vi "cdex - Initialize quadcopter 3D Model.vi"(8 "error in (no error)":errorcluster) -> (0 "error out":errorcluster, 3 "Main Scene Object":refnum<vi>)   [LabVIEW 2015]
uses:
  <vilib>/picture/3D Picture Control/Object/Create Object (drawable).vi
  <vilib>/picture/3D Picture Control/Object/Create Object (name).vi
  <vilib>/picture/3D Picture Control/Helpers/Apply Texture (no reference).vi
  <vilib>/picture/3D Picture Control/Object/Add Object (no reference).vi
  <vilib>/picture/3D Picture Control/Helpers/Set Clip Plane (no reference).vi
  <vilib>/picture/3D Picture Control/NI_3D Picture Control.lvlib
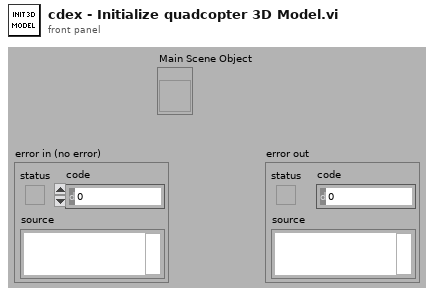
[diagram p1: front panel]
types:
  T1 = enum16{"As a Decal", "With Modulation", "With Blending", "As a replacement"}
  T2 = enum16{"Inherit Value", "No Culling", "Cull Back Face", "Cull Front Face", "Cull Both Faces"}
  T3 = enum16{"Normal Bin", "Opaque Bin", "Transparent Bin"}
  T4 = typedef "imagedata.ctl" = cluster{"image type":i32, "image depth":i32, "image":u8[], "mask":u8[], "colors":u32[], "Rectangle":cluster{"left":i16, "top":i16, "right":i16, "bottom":i16}}
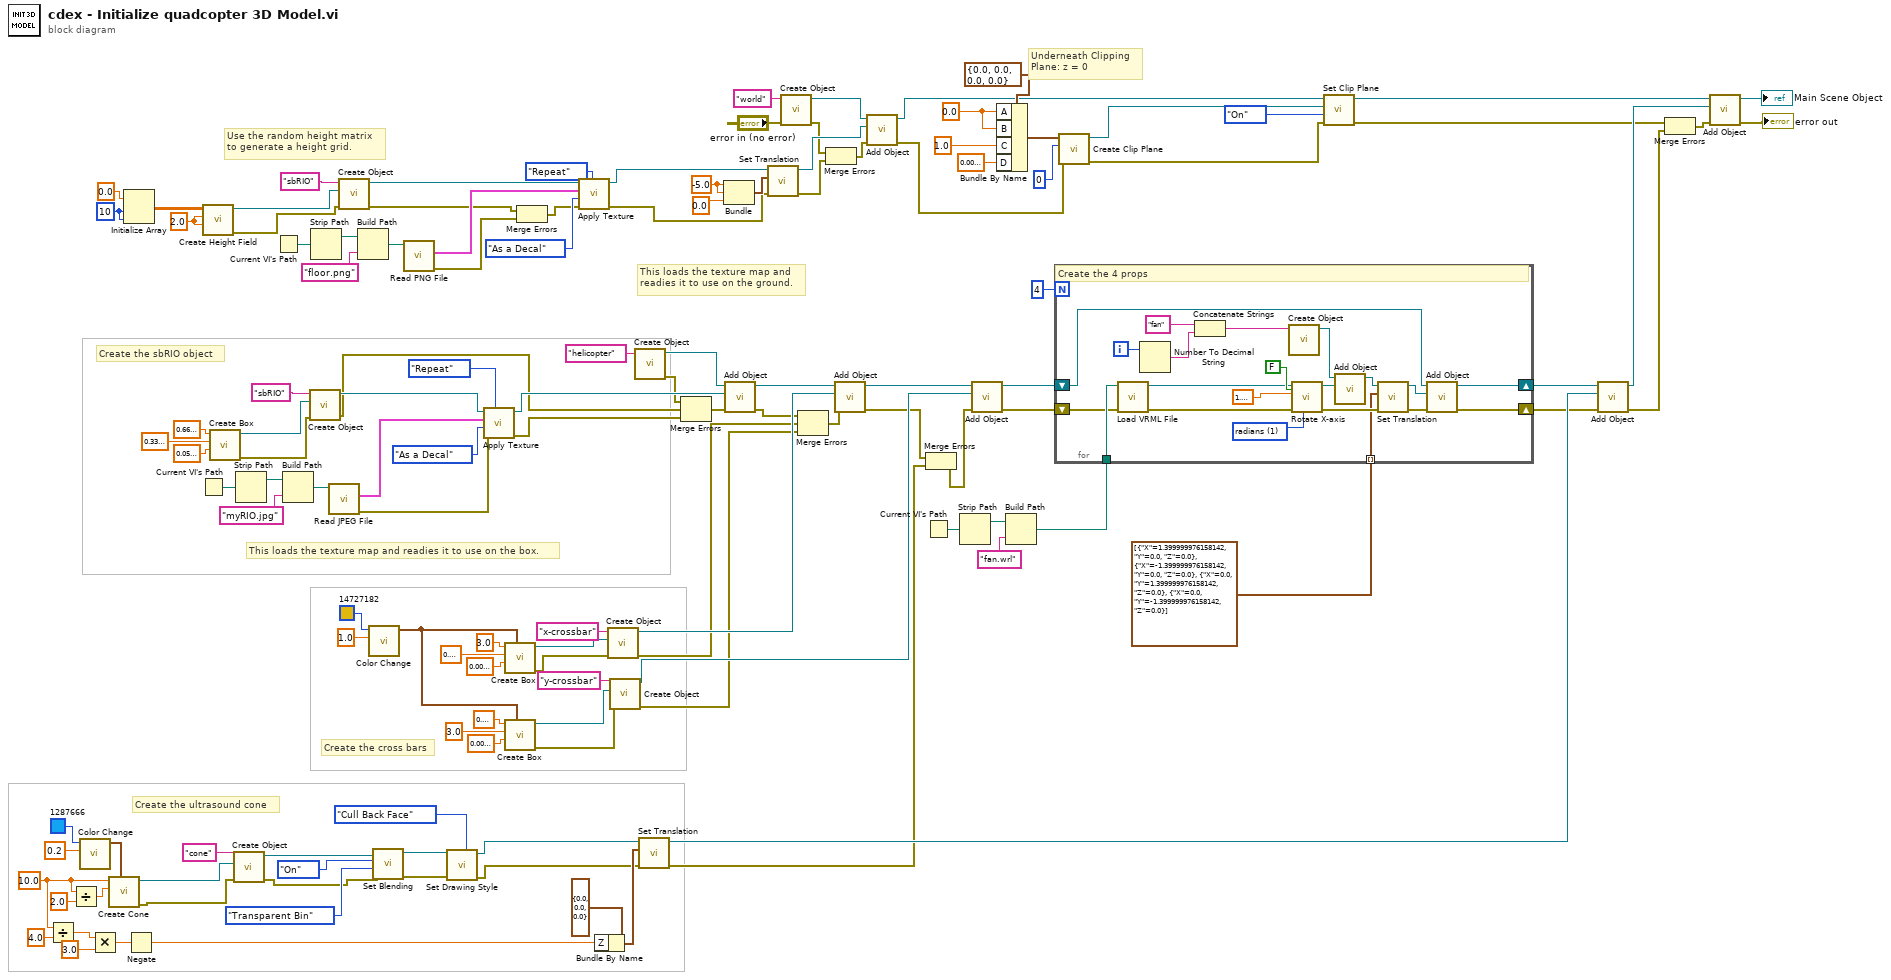
[diagram p0: block diagram]
diagram:
  w85 = 10 ("dimension size")
  w99 = sgl 0.0 ("A")
  w121 = sgl 10.0 ("Radius")
  w105 = sgl -5.0 ("y")
  w131 = sgl 2.0 ("Row Interval")
  # "This loads the texture map and\nreadies it to use on the ground."
  # "Underneath Clipping\nPlane: z = 0"
  # "Create the ultrasound cone"
  # "Create the cross bars"
  # "Create the sbRIO object"
  # "This loads the texture map and readies it to use on the box."
  # "Use the random height matrix\nto generate a height grid."
  n1 = Divide(x=w121, y=sgl 4.0) -> (x/y=w126:sgl)
  n2 = Divide(x=w121, y=sgl 2.0) -> (x/y=w122:sgl)
  n3 = call <vilib>:"Color Change.vi"("Alpha"=0.2, "Color"=u32 1287666) -> ("RGBA"=w118:cluster{"R":sgl, "G":sgl, "B":sgl, "A":sgl})  [unwired: 9 out]
  n4 = Multiply(x=w126, y=sgl 3.0) -> (x*y=w124:sgl)
  n5 = call <vilib>:"Create Cone.vi"("Color"=w118, "Radius"=w122, "Height"=w121) -> ("error out"=w44:errorcluster, "New Cone Refnum"=w64:refnum<vi>)  [unwired: 1 in, 6 out]
  n6 = Initialize Array(0.0 ("element"), w85, w85) -> (w83:dbl[][])
  n7 = Negate(x=w124) -> (-x=w128:sgl)
  n8 = Current VI's Path() -> (path=w104:path)
  n9 = call <vilib>:"Create Height Field.vi"("Column Interval"=w131, "Row Interval"=w131, "Data"=w83) -> ("error out"=w5:errorcluster, "New Height Field Refnum"=w56:refnum<vi>)  [unwired: 1 in, 6 out]
  n10 = call <vilib>:"Create Box.vi"("Length Z"=sgl 0.05, "Length Y"=sgl 0.33, "Length X"=sgl 0.66) -> ("error out"=w38:errorcluster, "New Box Refnum"=w78:refnum<vi>)  [unwired: 1 in, 6 out]
  n11 = call-poly <vilib>:"Create Object.vi"("error in (no error)"=w44, "Geometry"=w64, "Name"="cone") -> ("error out"=w43:errorcluster, "Scene:New Object"=w48:refnum<vi>)  [unwired: 7 in]
  n12 = Strip Path(path=w104) -> (stripped path=w103:path)  [unwired: 1 out]
  n13 = Current VI's Path() -> (path=w91:path)
  n14 = Build Path(base path=w103, name or relative path="myRIO.jpg") -> (appended path=w101:path)
  n15 = call-poly <vilib>:"Create Object.vi"("error in (no error)"=w38, "Geometry"=w78, "Name"="sbRIO") -> ("error out"=w35:errorcluster, "Scene:New Object"=w76:refnum<vi>)  [unwired: 7 in]
  n16 = Strip Path(path=w91) -> (stripped path=w92:path)  [unwired: 1 out]
  n17 = call <vilib>:"Read JPEG File.vi"("path to JPEG file"=w101) -> ("error out"=w37:errorcluster, "image data"=w72:T4)  [unwired: 1 in, 8 out]
  n18 = call-poly <vilib>:"Create Object.vi"("error in (no error)"=w5, "Geometry"=w56, "Name"="sbRIO") -> ("error out"=w6:errorcluster, "Scene:New Object"=w59:refnum<vi>)  [unwired: 7 in]
  n19 = Build Path(base path=w92, name or relative path="floor.png") -> (appended path=w94:path)
  n20 = call <vilib>:"Color Change.vi"("Alpha"=1.0, "Color"=u32 14727182) -> ("RGBA"=w100:cluster{"R":sgl, "G":sgl, "B":sgl, "A":sgl})  [unwired: 9 out]
  n21 = call <vilib>:"Set Blending.vi"("error in (no error)"=w43, "Bin"=T3."Transparent Bin" ("Blending:Bin"), "Mode"=enum16{"Inherit Value", "Off", "On"}."On" ("Blending:Mode"), "Scene Object In"=w48) -> ("error out"=w42:errorcluster, "Scene Object Out"=w47:refnum<vi>)  [unwired: 6 in]
  n22 = call <vilib>:"Read PNG File.vi"("path to PNG file"=w94) -> ("error out"=w8:errorcluster, "image data"=w57:T4)  [unwired: 1 in, 8 out]
  n23 = call <vilib>:"Set Drawing Style.vi"("Face Culling Mode"=T2."Cull Back Face" ("Draw Style:Face Culling Mode"), "error in (no error)"=w42, "Scene Object In"=w47) -> ("error out"=w41:errorcluster, "Scene Object Out"=w45:refnum<vi>)  [unwired: 7 in]
  n24 = call-poly <vilib>:"Apply Texture.vi"("Horizontal Wrap Mode"=enum16{"Clamp", "Repeat"}."Repeat", "error in (no error)"=w37, "Apply Mode"=T1."As a Decal", "Image Data"=w72, "Scene Object In"=w76) -> ("error out"=w36:errorcluster, "Scene Object Out"=w75:refnum<vi>)  [unwired: 5 in]
  n25 = call <vilib>:"Create Box.vi"("Color"=w100, "Length Z"=sgl 0.01, "Length Y"=sgl 0.1, "Length X"=sgl 3.0) -> ("error out"=w40:errorcluster, "New Box Refnum"=w71:refnum<vi>)  [unwired: 1 in, 5 out]
  n26 = call <vilib>:"Create Box.vi"("Color"=w100, "Length Z"=sgl 0.01, "Length Y"=sgl 3.0, "Length X"=sgl 0.1) -> ("error out"=w39:errorcluster, "New Box Refnum"=w68:refnum<vi>)  [unwired: 1 in, 5 out]
  n27 = Merge Errors(w6, w8) -> (w7:errorcluster)
  n28 = call-poly <vilib>:"Apply Texture.vi"("Horizontal Wrap Mode"=enum16{"Clamp", "Repeat"}."Repeat", "error in (no error)"=w7, "Apply Mode"=T1."As a Decal", "Image Data"=w57, "Scene Object In"=w59) -> ("error out"=w9:errorcluster, "Scene Object Out"=w61:refnum<vi>)  [unwired: 5 in]
  n29 = Bundle By Name(cluster=cluster{"X":sgl, "Y":sgl, "Z":sgl} {"X"=0.0, "Y"=0.0, "Z"=0.0} ("Translation"), "Z"=w128) -> (w130:cluster{"X":sgl, "Y":sgl, "Z":sgl})
  n30 = call-poly <vilib>:"Create Object.vi"("error in (no error)"=w40, "Geometry"=w71, "Name"="x-crossbar") -> ("error out"=w30:errorcluster, "Scene:New Object"=w70:refnum<vi>)  [unwired: 7 in]
  n31 = call-poly <vilib>:"Create Object.vi"("error in (no error)"=w39, "Geometry"=w68, "Name"="y-crossbar") -> ("error out"=w29:errorcluster, "Scene:New Object"=w67:refnum<vi>)  [unwired: 7 in]
  n32 = call-poly <vilib>:"Create Object.vi"("Name"="helicopter") -> ("error out"=w34:errorcluster, "Scene:New Object"=w82:refnum<vi>)  [unwired: 9 in]
  n33 = call <vilib>:"Set Translation.vi"("error in (no error)"=w41, "Translation"=w130, "Scene Object"=w45) -> ("error out"=w27:errorcluster, "Translated Object"=w54:refnum<vi>)  [unwired: 7 out]
  n34 = Merge Errors(w34, w35, w36) -> (w33:errorcluster)
  n35 = Bundle("y"=w105, "y"=w105, "-x"=0.0) -> (w117:cluster{"y":sgl, "y":sgl, "-x":dbl})  [unwired: 1 out]
  n36 = call-poly <vilib>:"Add Object.vi"("error in (no error)"=w33, "New Object In"=w75, "Scene Object In"=w82) -> ("error out"=w31:errorcluster, "Scene Object Out"=w81:refnum<vi>)  [unwired: 7 in]
  n37 = call <vilib>:"Set Translation.vi"("error in (no error)"=w9, "Translation"=w117, "Scene Object"=w61) -> ("error out"=w10:errorcluster, "Translated Object"=w23:refnum<vi>)  [unwired: 7 out]
  n38 = call-poly <vilib>:"Create Object.vi"("error in (no error)"="error in (no error)", "Name"="world") -> ("error out"=w12:errorcluster, "Scene:New Object"=w22:refnum<vi>)  [unwired: 8 in]
  n39 = Merge Errors(w31, w30, w29) -> (w32:errorcluster)
  n40 = Merge Errors(w12, w10) -> (w11:errorcluster)
  n41 = call-poly <vilib>:"Add Object.vi"("error in (no error)"=w32, "New Object In"=w70, "Scene Object In"=w81) -> ("error out"=w28:errorcluster, "Scene Object Out"=w80:refnum<vi>)  [unwired: 7 in]
  n42 = call-poly <vilib>:"Add Object.vi"("error in (no error)"=w11, "New Object In"=w23, "Scene Object In"=w22) -> ("error out"=w13:errorcluster, "Scene Object Out"=w21:refnum<vi>)  [unwired: 7 in]
  n43 = Current VI's Path() -> (path=w89:path)
  n44 = Merge Errors(w28, w27) -> (w26:errorcluster)
  n45 = Strip Path(path=w89) -> (stripped path=w88:path)  [unwired: 1 out]
  n46 = call-poly <vilib>:"Add Object.vi"("error in (no error)"=w26, "New Object In"=w67, "Scene Object In"=w80) -> ("error out"=w25:errorcluster, "Scene Object Out"=w79:refnum<vi>)  [unwired: 7 in]
  n47 = Bundle By Name(cluster=cluster{"A":sgl, "B":sgl, "C":sgl, "D":sgl} {"A"=0.0, "B"=0.0, "C"=0.0, "D"=0.0} ("Plane"), "A"=w99, "B"=w99, "C"=sgl 1.0 ("B"), "D"=sgl 0.01 ("B")) -> (w96:cluster{"A":sgl, "B":sgl, "C":sgl, "D":sgl})
  n48 = Build Path(base path=w88, name or relative path="fan.wrl") -> (appended path=w86:path)
  n49 = for {
    N: 4 -> [_]
    shift-right: [w151] -> w55
    shift-left: w79 -> [w152]
    tunnel: w86 -> [w153]
    shift-right: [w149] -> w24
    shift-left: w25 -> [w150]
    tunnel: cluster{"X":sgl, "Y":sgl, "Z":sgl}[] [{"X"=1.4, "Y"=0.0, "Z"=0.0}, {"X"=-1.4, "Y"=0.0, "Z"=0.0}, {"X"=0.0, "Y"=1.4, "Z"=0.0}, {"X"=0.0, "Y"=-1.4, "Z"=0.0}] -> [w142] mode=indexing
    i -> [w148]
    w141 = u16 1 items=["degree", "radians"] ("angle unit")
    # "Create the 4 props"
    n50 = call <vilib>:"Load VRML File.vi"("error in"=w150, "Path"=w153) -> ("error out"=w133:errorcluster, "Scene:Read Scene File"=w136:refnum<vi>)  [unwired: 8 out]
    n51 = Number To Decimal String(number=w148) -> (decimal integer string=w147:string)  [unwired: 1 in]
    n52 = Concatenate Strings("fan" ("string"), w147) -> (w146:string)
    n53 = call-poly <vilib>:"Create Object.vi"("Name"=w146) -> ("Scene:New Object"=w138:refnum<vi>)  [unwired: 9 in, 1 out]
    n54 = call <vilib>:"Rotate X-axis.vi"("angle unit"=w141, "Relative?"=FALSE, "error in (no error)"=w133, "angle"=1.5707963267948966, "Scene Object In"=w136) -> ("error out"=w143:errorcluster, "Scene Object Out"=w135:refnum<vi>)  [unwired: 5 in]
    n55 = call-poly <vilib>:"Add Object.vi"("New Object In"=w135, "Scene Object In"=w138) -> ("Scene Object Out"=w134:refnum<vi>)  [unwired: 8 in, 1 out]
    n56 = call <vilib>:"Set Translation.vi"("error in (no error)"=w143, "Translation"=w142, "Scene Object"=w134) -> ("error out"=w139:errorcluster, "Translated Object"=w137:refnum<vi>)  [unwired: 7 in]
    n57 = call-poly <vilib>:"Add Object.vi"("error in (no error)"=w139, "New Object In"=w137, "Scene Object In"=w152) -> ("error out"=w149:errorcluster, "Scene Object Out"=w151:refnum<vi>)  [unwired: 7 in]
  }
  n58 = call <vilib>:"Create Clip Plane.vi"("error in (no error)"=w13, "Number"=0, "Plane"=w96) -> ("error out"=w14:errorcluster, "New Clip Plane Refnum"=w20:refnum<vi>)  [unwired: 7 out]
  n59 = call-poly <vilib>:"Set Clip Plane.vi"("error in (no error)"=w14, "Clip Plane State"=enum16{"Inherit Value", "Off", "On"}."On", "Clip Plane Refnum In"=w20, "Scene Object In"=w21) -> ("error out"=w15:errorcluster, "Scene Object Out"=w18:refnum<vi>)  [unwired: 6 in]
  n60 = call-poly <vilib>:"Add Object.vi"("error in (no error)"=w24, "New Object In"=w54, "Scene Object In"=w55) -> ("error out"=w17:errorcluster, "Scene Object Out"=w53:refnum<vi>)  [unwired: 7 in]
  n61 = Merge Errors(w15, w17) -> (w16:errorcluster)
  n62 = call-poly <vilib>:"Add Object.vi"("error in (no error)"=w16, "New Object In"=w53, "Scene Object In"=w18) -> ("error out"=→"error out":errorcluster, "Scene Object Out"=→"Main Scene Object":refnum<vi>)  [unwired: 7 in]
